vi "Untitled 3.vi"() -> ()   [LabVIEW 2016]
uses:
  <vilib>/NXT/Block Support/NXT_InputPort.ctl
  <vilib>/NXT/Dual Mode Library/Waits/Wait_Bump.vi
  <vilib>/NXT/NXTIO Xnodes/NXTIONodeSubVIs/LEGOMoveAllMotors.vi
  <vilib>/NXT/NXTIO Xnodes/NXTIOXNode/NXTIO.xnode
  <vilib>/NXT/Subs/LVHSConnector.ctl
  <vilib>/NXT/LegoClasses/BrickReference/BrickReference.lvclass
panel:
  out "Array":dbl[](array[numeric])
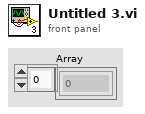
[diagram p1: front panel]
types:
  T1 = typedef "NXT_InputPort.ctl" = u32
  T2 = typedef "LVHSConnector.ctl" = refnum<class "BrickReference.lvclass">
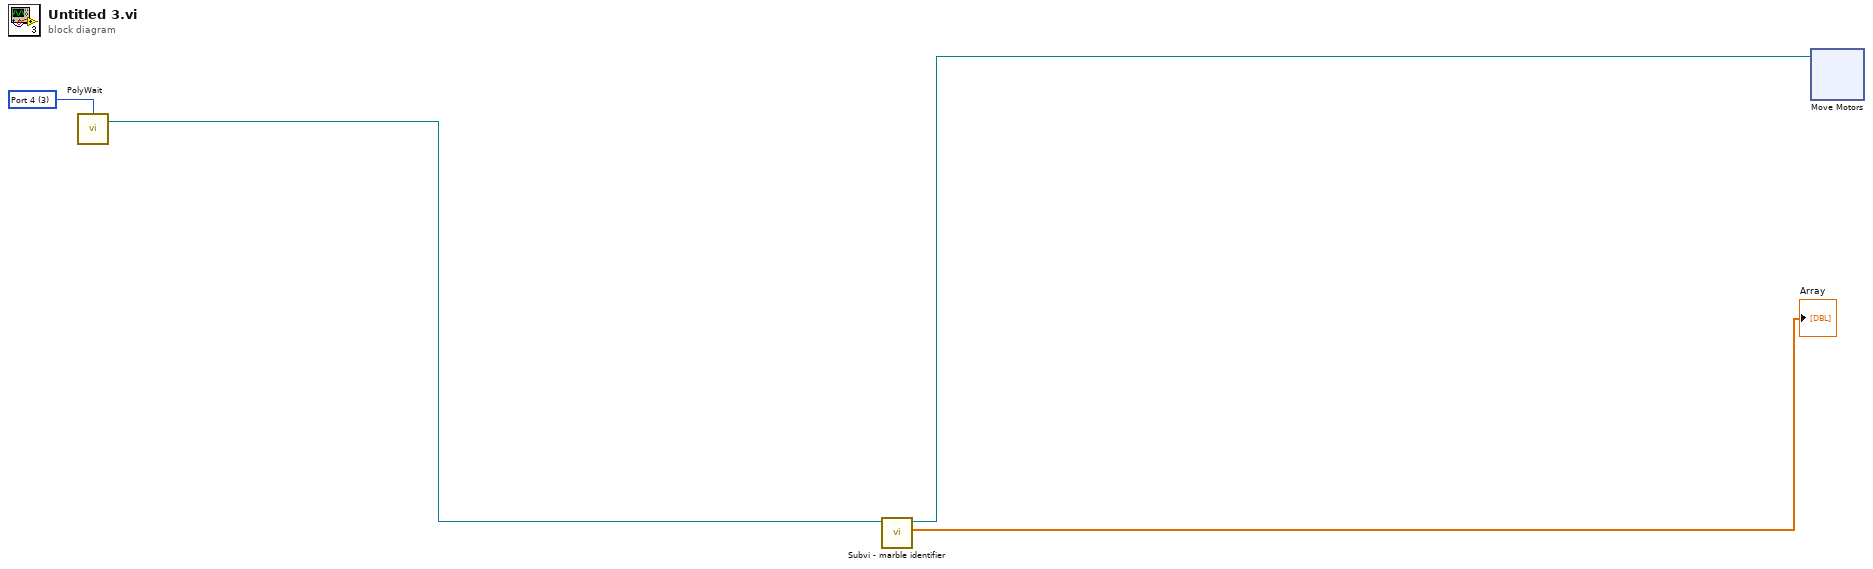
[diagram p0: block diagram]
diagram:
  w3 = T1 3 items=["Port 1", "Port 2", "Port 3", "Port 4"] ("Port (Port 1)")
  n1 = call-poly <vilib>:"PolyWait.vi"("Port (Port 1)"=w3) -> ("NXT/EV3"=w4:T2)  [unwired: 3 in]
  n2 = call "Subvi - marble identifier.vi"("BrickReference in"=w4) -> ("Array"=→"Array":dbl[], "BrickReference out"=w1:T2)  [unwired: 9 in]
  n3 = xnode "Move Motors"("NXT/EV3"=w1) -> ()  [unwired: 2 in, 1 out]
